vi "Lab Panel V5.10.vi"() -> ()   [LabVIEW 2013] (continued)
                    n2520 = local read "SET LAB01-1"() -> (w4770:T5)
                    n2521 = local read "DISP LAB01-1"() -> (w4771:T4)
                    n2522 = local read "SIG LAB01-1"() -> (w4775:T2)
                    n2523 = Bundle("FAIL LAB01-1"=w4766, "SIG LAB01-1"=w4775, "TEMP START LAB01-1"=w4774, "DISP LAB01-1"=w4771, "SET LAB01-1"=w4770, "TDMS LAB01-1"=w4773) -> (w4760:T32)  [unwired: 1 in]
                    n2524 = call "sub vi - cycle&temp fail v7.vi"("Amps Lo?"=w4772, "Input Cluster"=w4760, "SELECT"=w4769, "Amps Hi?"=w4768, "Result In"=w4763) -> ("(FAIL) out"=w4765:cluster{"FAIL LO":dbl, "FAIL HI":dbl}, "(DISP) out"=w4761:T4, "T-RISE"=w4762:cluster{"T-RISE (L)":dbl, "T-RISE (N)":dbl}, "Result Out"=w4764:bool, "file error"=w4767:errorcluster)  [unwired: 10 in]
                    n2525 = local write "TEMP RISE LAB01-1"(w4762) -> ()
                    n2526 = local write "FAIL LAB01-1"(w4765) -> ()
                    n2527 = local write "DISP LAB01-1"(w4761) -> ()
                    n2528 = local write "RESULT LAB01-1"(w4764) -> ()
                    n2529 = local write "data file error"(w4767) -> ()
                  }
                }
              }
              frame #1 {
                # "LAB01-2"
                n2530 = case shown="True" w4777 {
                  tunnel: w4779 -> [_ w4792]
                  tunnel: w4776 -> [_ w4789]
                  tunnel: w4778 -> [_ w4788]
                  frame False {
                  }
                  frame True {
                    n2531 = local read "TEMP START LAB01-2"() -> (w4794:cluster{"TL":dbl, "TN":dbl})
                    n2532 = local read "FAIL LAB01-2"() -> (w4785:cluster{"LO":dbl, "HI":dbl})
                    n2533 = local read "TDMS LAB01-2"() -> (w4793:refnum<k34>)
                    n2534 = local read "SET LAB01-2"() -> (w4790:T5)
                    n2535 = local read "DISP LAB01-2"() -> (w4791:T4)
                    n2536 = local read "RESULT LAB01-2"() -> (w4782:bool)
                    n2537 = local read "SIG LAB01-2"() -> (w4795:T2)
                    n2538 = Bundle("FAIL LAB01-2"=w4785, "SIG LAB01-2"=w4795, "TEMP START LAB01-2"=w4794, "DISP LAB01-2"=w4791, "SET LAB01-2"=w4790, "TDMS LAB01-2"=w4793) -> (w4780:T33)  [unwired: 1 in]
                    n2539 = call "sub vi - cycle&temp fail v7.vi"("Amps Lo?"=w4792, "Input Cluster"=w4780, "SELECT"=w4789, "Amps Hi?"=w4788, "Result In"=w4782) -> ("(FAIL) out"=w4784:cluster{"FAIL LO":dbl, "FAIL HI":dbl}, "(DISP) out"=w4787:T4, "T-RISE"=w4781:cluster{"T-RISE (L)":dbl, "T-RISE (N)":dbl}, "Result Out"=w4783:bool, "file error"=w4786:errorcluster)  [unwired: 10 in]
                    n2540 = local write "TEMP RISE LAB01-2"(w4781) -> ()
                    n2541 = local write "FAIL LAB01-2"(w4784) -> ()
                    n2542 = local write "DISP LAB01-2"(w4787) -> ()
                    n2543 = local write "RESULT LAB01-2"(w4783) -> ()
                    n2544 = local write "data file error"(w4786) -> ()
                  }
                }
              }
              frame #2 {
                # "LAB02-1"
                n2545 = case shown="True" w4797 {
                  tunnel: w4799 -> [_ w4812]
                  tunnel: w4796 -> [_ w4809]
                  tunnel: w4798 -> [_ w4808]
                  frame False {
                  }
                  frame True {
                    n2546 = local read "TEMP START LAB02-1"() -> (w4814:cluster{"TL":dbl, "TN":dbl})
                    n2547 = local read "FAIL LAB02-1"() -> (w4805:cluster{"LO":dbl, "HI":dbl})
                    n2548 = local read "TDMS LAB02-1"() -> (w4813:refnum<k34>)
                    n2549 = local read "SET LAB02-1"() -> (w4810:T5)
                    n2550 = local read "DISP LAB02-1"() -> (w4811:T4)
                    n2551 = local read "SIG LAB02-1"() -> (w4815:T2)
                    n2552 = local read "RESULT LAB02-1"() -> (w4802:bool)
                    n2553 = Bundle("FAIL LAB02-1"=w4805, "SIG LAB02-1"=w4815, "TEMP START LAB02-1"=w4814, "DISP LAB02-1"=w4811, "SET LAB02-1"=w4810, "TDMS LAB02-1"=w4813) -> (w4800:T34)  [unwired: 1 in]
                    n2554 = call "sub vi - cycle&temp fail v7.vi"("Amps Lo?"=w4812, "Input Cluster"=w4800, "SELECT"=w4809, "Amps Hi?"=w4808, "Result In"=w4802) -> ("(FAIL) out"=w4804:cluster{"FAIL LO":dbl, "FAIL HI":dbl}, "(DISP) out"=w4807:T4, "T-RISE"=w4801:cluster{"T-RISE (L)":dbl, "T-RISE (N)":dbl}, "Result Out"=w4803:bool, "file error"=w4806:errorcluster)  [unwired: 10 in]
                    n2555 = local write "TEMP RISE LAB02-1"(w4801) -> ()
                    n2556 = local write "FAIL LAB02-1"(w4804) -> ()
                    n2557 = local write "DISP LAB02-1"(w4807) -> ()
                    n2558 = local write "RESULT LAB02-1"(w4803) -> ()
                    n2559 = local write "data file error"(w4806) -> ()
                  }
                }
              }
              frame #3 {
                # "LAB02-2"
                n2560 = case shown="True" w4817 {
                  tunnel: w4819 -> [_ w4832]
                  tunnel: w4816 -> [_ w4829]
                  tunnel: w4818 -> [_ w4828]
                  frame False {
                  }
                  frame True {
                    n2561 = local read "TEMP START LAB02-2"() -> (w4834:cluster{"TL":dbl, "TN":dbl})
                    n2562 = local read "FAIL LAB02-2"() -> (w4825:cluster{"LO":dbl, "HI":dbl})
                    n2563 = local read "TDMS LAB02-2"() -> (w4833:refnum<k34>)
                    n2564 = local read "SET LAB02-2"() -> (w4830:T5)
                    n2565 = local read "DISP LAB02-2"() -> (w4831:T4)
                    n2566 = local read "SIG LAB02-2"() -> (w4835:T2)
                    n2567 = local read "RESULT LAB02-2"() -> (w4822:bool)
                    n2568 = Bundle("FAIL LAB02-2"=w4825, "SIG LAB02-2"=w4835, "TEMP START LAB02-2"=w4834, "DISP LAB02-2"=w4831, "SET LAB02-2"=w4830, "TDMS LAB02-2"=w4833) -> (w4820:T35)  [unwired: 1 in]
                    n2569 = call "sub vi - cycle&temp fail v7.vi"("Amps Lo?"=w4832, "Input Cluster"=w4820, "SELECT"=w4829, "Amps Hi?"=w4828, "Result In"=w4822) -> ("(FAIL) out"=w4824:cluster{"FAIL LO":dbl, "FAIL HI":dbl}, "(DISP) out"=w4827:T4, "T-RISE"=w4821:cluster{"T-RISE (L)":dbl, "T-RISE (N)":dbl}, "Result Out"=w4823:bool, "file error"=w4826:errorcluster)  [unwired: 10 in]
                    n2570 = local write "TEMP RISE LAB02-2"(w4821) -> ()
                    n2571 = local write "FAIL LAB02-2"(w4824) -> ()
                    n2572 = local write "DISP LAB02-2"(w4827) -> ()
                    n2573 = local write "RESULT LAB02-2"(w4823) -> ()
                    n2574 = local write "data file error"(w4826) -> ()
                  }
                }
              }
              frame #4 {
                # "LAB03-1"
                n2575 = case shown="True" w4837 {
                  tunnel: w4839 -> [_ w4852]
                  tunnel: w4836 -> [_ w4849]
                  tunnel: w4838 -> [_ w4848]
                  frame False {
                  }
                  frame True {
                    n2576 = local read "TEMP START LAB03-1"() -> (w4854:cluster{"TL":dbl, "TN":dbl})
                    n2577 = local read "FAIL LAB03-1"() -> (w4845:cluster{"LO":dbl, "HI":dbl})
                    n2578 = local read "TDMS LAB03-1"() -> (w4853:refnum<k34>)
                    n2579 = local read "SET LAB03-1"() -> (w4850:T5)
                    n2580 = local read "DISP LAB03-1"() -> (w4851:T4)
                    n2581 = local read "SIG LAB03-1"() -> (w4855:T2)
                    n2582 = local read "RESULT LAB03-1"() -> (w4842:bool)
                    n2583 = Bundle("FAIL LAB03-1"=w4845, "SIG LAB03-1"=w4855, "TEMP START LAB03-1"=w4854, "DISP LAB03-1"=w4851, "SET LAB03-1"=w4850, "TDMS LAB03-1"=w4853) -> (w4840:T36)  [unwired: 1 in]
                    n2584 = call "sub vi - cycle&temp fail v7.vi"("Amps Lo?"=w4852, "Input Cluster"=w4840, "SELECT"=w4849, "Amps Hi?"=w4848, "Result In"=w4842) -> ("(FAIL) out"=w4844:cluster{"FAIL LO":dbl, "FAIL HI":dbl}, "(DISP) out"=w4847:T4, "T-RISE"=w4841:cluster{"T-RISE (L)":dbl, "T-RISE (N)":dbl}, "Result Out"=w4843:bool, "file error"=w4846:errorcluster)  [unwired: 10 in]
                    n2585 = local write "TEMP RISE LAB03-1"(w4841) -> ()
                    n2586 = local write "FAIL LAB03-1"(w4844) -> ()
                    n2587 = local write "DISP LAB03-1"(w4847) -> ()
                    n2588 = local write "RESULT LAB03-1"(w4843) -> ()
                    n2589 = local write "data file error"(w4846) -> ()
                  }
                }
              }
              frame #5 {
                # "LAB03-2"
                n2590 = case shown="True" w4857 {
                  tunnel: w4859 -> [_ w4872]
                  tunnel: w4856 -> [_ w4869]
                  tunnel: w4858 -> [_ w4868]
                  frame False {
                  }
                  frame True {
                    n2591 = local read "TEMP START LAB03-2"() -> (w4874:cluster{"TL":dbl, "TN":dbl})
                    n2592 = local read "FAIL LAB03-2"() -> (w4865:cluster{"LO":dbl, "HI":dbl})
                    n2593 = local read "TDMS LAB03-2"() -> (w4873:refnum<k34>)
                    n2594 = local read "SET LAB03-2"() -> (w4870:T5)
                    n2595 = local read "DISP LAB03-2"() -> (w4871:T4)
                    n2596 = local read "RESULT LAB03-2"() -> (w4862:bool)
                    n2597 = local read "SIG LAB03-2"() -> (w4875:T2)
                    n2598 = Bundle("FAIL LAB03-2"=w4865, "SIG LAB03-2"=w4875, "TEMP START LAB03-2"=w4874, "DISP LAB03-2"=w4871, "SET LAB03-2"=w4870, "TDMS LAB03-2"=w4873) -> (w4860:T37)  [unwired: 1 in]
                    n2599 = call "sub vi - cycle&temp fail v7.vi"("Amps Lo?"=w4872, "Input Cluster"=w4860, "SELECT"=w4869, "Amps Hi?"=w4868, "Result In"=w4862) -> ("(FAIL) out"=w4864:cluster{"FAIL LO":dbl, "FAIL HI":dbl}, "(DISP) out"=w4867:T4, "T-RISE"=w4861:cluster{"T-RISE (L)":dbl, "T-RISE (N)":dbl}, "Result Out"=w4863:bool, "file error"=w4866:errorcluster)  [unwired: 10 in]
                    n2600 = local write "FAIL LAB03-2"(w4864) -> ()
                    n2601 = local write "TEMP RISE LAB03-2"(w4861) -> ()
                    n2602 = local write "DISP LAB03-2"(w4867) -> ()
                    n2603 = local write "RESULT LAB03-2"(w4863) -> ()
                    n2604 = local write "data file error"(w4866) -> ()
                  }
                }
              }
              frame #6 {
                # "LAB04-1"
                n2605 = case shown="True" w4877 {
                  tunnel: w4879 -> [_ w4892]
                  tunnel: w4876 -> [_ w4889]
                  tunnel: w4878 -> [_ w4888]
                  frame False {
                  }
                  frame True {
                    n2606 = local read "TEMP START LAB04-1"() -> (w4894:cluster{"TL":dbl, "TN":dbl})
                    n2607 = local read "FAIL LAB04-1"() -> (w4885:cluster{"LO":dbl, "HI":dbl})
                    n2608 = local read "TDMS LAB04-1"() -> (w4893:refnum<k34>)
                    n2609 = local read "SET LAB04-1"() -> (w4890:T5)
                    n2610 = local read "DISP LAB04-1"() -> (w4891:T4)
                    n2611 = local read "SIG LAB04-1"() -> (w4895:T2)
                    n2612 = local read "RESULT LAB04-1"() -> (w4882:bool)
                    n2613 = Bundle("FAIL LAB04-1"=w4885, "SIG LAB04-1"=w4895, "TEMP START LAB04-1"=w4894, "DISP LAB04-1"=w4891, "SET LAB04-1"=w4890, "TDMS LAB04-1"=w4893) -> (w4880:T38)  [unwired: 1 in]
                    n2614 = call "sub vi - cycle&temp fail v7.vi"("Amps Lo?"=w4892, "Input Cluster"=w4880, "SELECT"=w4889, "Amps Hi?"=w4888, "Result In"=w4882) -> ("(FAIL) out"=w4884:cluster{"FAIL LO":dbl, "FAIL HI":dbl}, "(DISP) out"=w4887:T4, "T-RISE"=w4881:cluster{"T-RISE (L)":dbl, "T-RISE (N)":dbl}, "Result Out"=w4883:bool, "file error"=w4886:errorcluster)  [unwired: 10 in]
                    n2615 = local write "TEMP RISE LAB04-1"(w4881) -> ()
                    n2616 = local write "FAIL LAB04-1"(w4884) -> ()
                    n2617 = local write "DISP LAB04-1"(w4887) -> ()
                    n2618 = local write "RESULT LAB04-1"(w4883) -> ()
                    n2619 = local write "data file error"(w4886) -> ()
                  }
                }
              }
              frame #7 {
                # "LAB04-2"
                n2620 = case shown="True" w4897 {
                  tunnel: w4899 -> [_ w4912]
                  tunnel: w4896 -> [_ w4909]
                  tunnel: w4898 -> [_ w4908]
                  frame False {
                  }
                  frame True {
                    n2621 = local read "TEMP START LAB04-2"() -> (w4914:cluster{"TL":dbl, "TN":dbl})
                    n2622 = local read "FAIL LAB04-2"() -> (w4905:cluster{"LO":dbl, "HI":dbl})
                    n2623 = local read "TDMS LAB04-2"() -> (w4913:refnum<k34>)
                    n2624 = local read "SET LAB04-2"() -> (w4910:T5)
                    n2625 = local read "DISP LAB04-2"() -> (w4911:T4)
                    n2626 = local read "SIG LAB04-2"() -> (w4915:T2)
                    n2627 = local read "RESULT LAB04-2"() -> (w4902:bool)
                    n2628 = Bundle("FAIL LAB04-2"=w4905, "SIG LAB04-2"=w4915, "TEMP START LAB04-2"=w4914, "DISP LAB04-2"=w4911, "SET LAB04-2"=w4910, "TDMS LAB04-2"=w4913) -> (w4900:T39)  [unwired: 1 in]
                    n2629 = call "sub vi - cycle&temp fail v7.vi"("Amps Lo?"=w4912, "Input Cluster"=w4900, "SELECT"=w4909, "Amps Hi?"=w4908, "Result In"=w4902) -> ("(FAIL) out"=w4904:cluster{"FAIL LO":dbl, "FAIL HI":dbl}, "(DISP) out"=w4907:T4, "T-RISE"=w4901:cluster{"T-RISE (L)":dbl, "T-RISE (N)":dbl}, "Result Out"=w4903:bool, "file error"=w4906:errorcluster)  [unwired: 10 in]
                    n2630 = local write "TEMP RISE LAB04-2"(w4901) -> ()
                    n2631 = local write "FAIL LAB04-2"(w4904) -> ()
                    n2632 = local write "DISP LAB04-2"(w4907) -> ()
                    n2633 = local write "RESULT LAB04-2"(w4903) -> ()
                    n2634 = local write "data file error"(w4906) -> ()
                  }
                }
              }
              frame #8 {
                # "LAB05-1"
                n2635 = case shown="True" w4917 {
                  tunnel: w4919 -> [_ w4932]
                  tunnel: w4916 -> [_ w4929]
                  tunnel: w4918 -> [_ w4928]
                  frame False {
                  }
                  frame True {
                    n2636 = local read "TEMP START LAB05-1"() -> (w4934:cluster{"TL":dbl, "TN":dbl})
                    n2637 = local read "FAIL LAB05-1"() -> (w4925:cluster{"LO":dbl, "HI":dbl})
                    n2638 = local read "TDMS LAB05-1"() -> (w4933:refnum<k34>)
                    n2639 = local read "SET LAB05-1"() -> (w4930:T5)
                    n2640 = local read "DISP LAB05-1"() -> (w4931:T4)
                    n2641 = local read "SIG LAB05-1"() -> (w4935:T2)
                    n2642 = local read "RESULT LAB05-1"() -> (w4922:bool)
                    n2643 = Bundle("FAIL LAB05-1"=w4925, "SIG LAB05-1"=w4935, "TEMP START LAB05-1"=w4934, "DISP LAB05-1"=w4931, "SET LAB05-1"=w4930, "TDMS LAB05-1"=w4933) -> (w4920:T40)  [unwired: 1 in]
                    n2644 = call "sub vi - cycle&temp fail v7.vi"("Amps Lo?"=w4932, "Input Cluster"=w4920, "SELECT"=w4929, "Amps Hi?"=w4928, "Result In"=w4922) -> ("(FAIL) out"=w4924:cluster{"FAIL LO":dbl, "FAIL HI":dbl}, "(DISP) out"=w4927:T4, "T-RISE"=w4921:cluster{"T-RISE (L)":dbl, "T-RISE (N)":dbl}, "Result Out"=w4923:bool, "file error"=w4926:errorcluster)  [unwired: 10 in]
                    n2645 = local write "TEMP RISE LAB05-1"(w4921) -> ()
                    n2646 = local write "FAIL LAB05-1"(w4924) -> ()
                    n2647 = local write "DISP LAB05-1"(w4927) -> ()
                    n2648 = local write "RESULT LAB05-1"(w4923) -> ()
                    n2649 = local write "data file error"(w4926) -> ()
                  }
                }
              }
              frame #9 {
                # "LAB05-2"
                n2650 = case shown="True" w4937 {
                  tunnel: w4939 -> [_ w4952]
                  tunnel: w4936 -> [_ w4949]
                  tunnel: w4938 -> [_ w4948]
                  frame False {
                  }
                  frame True {
                    n2651 = local read "TEMP START LAB05-2"() -> (w4954:cluster{"TL":dbl, "TN":dbl})
                    n2652 = local read "FAIL LAB05-2"() -> (w4945:cluster{"LO":dbl, "HI":dbl})
                    n2653 = local read "TDMS LAB05-2"() -> (w4953:refnum<k34>)
                    n2654 = local read "SET LAB05-2"() -> (w4950:T5)
                    n2655 = local read "DISP LAB05-2"() -> (w4951:T4)
                    n2656 = local read "SIG LAB05-2"() -> (w4955:T2)
                    n2657 = local read "RESULT LAB05-2"() -> (w4942:bool)
                    n2658 = Bundle("FAIL LAB05-2"=w4945, "SIG LAB05-2"=w4955, "TEMP START LAB05-2"=w4954, "DISP LAB05-2"=w4951, "SET LAB05-2"=w4950, "TDMS LAB05-2"=w4953) -> (w4940:T41)  [unwired: 1 in]
                    n2659 = call "sub vi - cycle&temp fail v7.vi"("Amps Lo?"=w4952, "Input Cluster"=w4940, "SELECT"=w4949, "Amps Hi?"=w4948, "Result In"=w4942) -> ("(FAIL) out"=w4944:cluster{"FAIL LO":dbl, "FAIL HI":dbl}, "(DISP) out"=w4947:T4, "T-RISE"=w4941:cluster{"T-RISE (L)":dbl, "T-RISE (N)":dbl}, "Result Out"=w4943:bool, "file error"=w4946:errorcluster)  [unwired: 10 in]
                    n2660 = local write "TEMP RISE LAB05-2"(w4941) -> ()
                    n2661 = local write "FAIL LAB05-2"(w4944) -> ()
                    n2662 = local write "DISP LAB05-2"(w4947) -> ()
                    n2663 = local write "RESULT LAB05-2"(w4943) -> ()
                    n2664 = local write "data file error"(w4946) -> ()
                  }
                }
              }
            }
          }
          frame #15 {
            # "run calibration routine"
            n2665 = local read "SET (cal)"() -> (w4956:bool)
            n2666 = case shown="True" w4956 {
              frame False {
              }
              frame True {
                n2667 = stacked-sequence {
                  seq-local: [w4957 _ _] -> [_ w4959 _]
                  frame #0 {
                    n2668 = call "CALIBRATION PASSWORD"() -> ("PASSWORD"=w4957:string)  [unwired: 17 in, 2 out]
                  }
                  frame #1 {
                    n2669 = Equal?(x=w4959, y="7777") -> (x = y?=w4958:bool)
                    n2670 = case shown="True" w4958 {
                      frame False {
                      }
                      frame True {
                        n2671 = stacked-sequence {
                          frame #0 {
                            n2672 = local read "Temp Test Cal"() -> (w4961:dbl)
                            n2673 = call "sub vi - calibration v1.vi"("Temp Test Cal"=w4961) -> ()  [unwired: 11 in]
                          }
                          frame #1 {
                            n2674 = call "sub vi - get calibration values v1.vi"() -> ("TEMP REF CAL"=w4962:dbl, "LAB01 (CAL)"=w4967:T14, "LAB02 (CAL)"=w4966:T15, "LAB03 (CAL)"=w4965:T14, "LAB04 (CAL)"=w4964:T14, "calibration file error out"=w4968:errorcluster, "LAB05 (CAL)"=w4963:T14)  [unwired: 9 in]
                            n2675 = local write "TEMP REF cal"(w4962) -> ()
                            n2676 = local write "cal file error out"(w4968) -> ()
                            n2677 = local write "CAL LAB04"(w4964) -> ()
                            n2678 = local write "CAL LAB05"(w4963) -> ()
                            n2679 = local write "CAL LAB01"(w4967) -> ()
                            n2680 = local write "CAL LAB02"(w4966) -> ()
                            n2681 = local write "CAL LAB03"(w4965) -> ()
                          }
                        }
                      }
                    }
                  }
                  frame #2 {
                    n2682 = local write "SET (cal)"(FALSE) -> ()
                  }
                }
              }
            }
          }
          frame #16 {
            # "save certain settings to file"
            n2683 = String To Path(string="c:\\crabtree\\Set Up\\") -> (path=w4971:path)
            n2684 = Build Path(base path=w4971, name or relative path="settings.bin") -> (appended path=w4973:path)
            n2685 = Build Path(base path=w4971, name or relative path="mail.bin") -> (appended path=w4970:path)
            n2686 = Create Folder(path (use dialog)=w4971) -> (error out=w4976:errorcluster)  [unwired: 2 in, 2 out]
            n2687 = call <vilib>:"Clear Errors.vi"("error in (no error)"=w4976) -> ()  [unwired: 6 in, 1 out]
            n2688 = stacked-sequence {
              seq-local: [w4988 _] -> [_ w5001]
              tunnel: w4973 -> [_ w5002]
              tunnel: w4970 -> [_ w5000]
              frame #0 {
                n2689 = local read "C drive data root dir"() -> (w4987:path)
                n2690 = local read "Select COM port"() -> (w4984:refnum<visa-resource-name>)
                n2691 = local read "Network Directory"() -> (w4993:path)
                n2692 = local read "SET LAB05-2"() -> (w4992:T5)
                n2693 = local read "SET LAB05-1"() -> (w4991:T5)
                n2694 = local read "SET LAB04-2"() -> (w4990:T5)
                n2695 = local read "SET LAB03-2"() -> (w4994:T5)
                n2696 = local read "SET LAB04-1"() -> (w4989:T5)
                n2697 = local read "SET LAB03-1"() -> (w4995:T5)
                n2698 = local read "SET LAB02-2"() -> (w4996:T5)
                n2699 = local read "SET LAB02-1"() -> (w4997:T5)
                n2700 = local read "Temp Delay Lps"() -> (w4983:dbl)
                n2701 = local read "Amps Fail level"() -> (w4979:dbl)
                n2702 = local read "SET LAB01-2"() -> (w4998:T5)
                n2703 = local read "Temp Test Cal"() -> (w4980:dbl)
                n2704 = local read "SET LAB01-1"() -> (w4999:T5)
                n2705 = local read "Mail Test File To:"() -> (w4978:string)
                n2706 = local read "Temp Value"() -> (w4982:dbl)
                n2707 = local read "Fail Loops"() -> (w4981:dbl)
                n2708 = local read "Mail Test Fail"() -> (w4977:bool)
                n2709 = local read "RATE (Hz)"() -> (w4986:dbl)
                n2710 = local read "SAMPLES"() -> (w4985:dbl)
                n2711 = Bundle("SET LAB01-1"=w4999, "SET LAB01-2"=w4998, "SET LAB02-1"=w4997, "SET LAB02-2"=w4996, "SET LAB03-1"=w4995, "SET LAB03-2"=w4994, "SET LAB04-1"=w4989, "SET LAB04-2"=w4990, "SET LAB05-1"=w4991, "SET LAB05-2"=w4992, "Network Directory"=w4993, "C drive data root dir"=w4987, "RATE (Hz)"=w4986, "SAMPLES"=w4985, "Select COM port"=w4984, "Temp Delay Lps"=w4983, "Temp Value"=w4982, "Fail Loops"=w4981, "Temp Test Cal"=w4980, "Amps Fail level"=w4979, "Mail Test File To:"=w4978, "Mail Test Fail"=w4977) -> (w4988:T22)  [unwired: 1 in]
              }
              frame #1 {
                n2712 = event shown="[1] \"SET LAB01-1\", \"SET LAB01-2\", \"SET LAB02-1\", \"SET LAB02-2\", \"SET LAB03-1\", \"SET LAB03-2\", \"SET LAB04-1\", \"SET LAB04-2\", \"SET LAB05-1\", \"SET LAB05-2\", \"Network Directory\", \"C drive data root dir\", \"RATE (Hz)\", \"SAMPLES\", \"Select COM port\", \"Temp Delay Lps\", \"Temp Value\", \"Fail Loops\", \"Temp Test Cal\", \"Amps Fail level\", \"Mail Test File To:\", \"Mail Test Fail\": Value Change" {
                  selector: _ -> [_ _ _]
                  dyn-events: _ -> [_ _ _]
                  timeout: 10.0 -> [_ _ _]
                  tunnel: w5002 -> [_ w5004 _]
                  tunnel: w5001 -> [_ w5005 _]
                  tunnel: w5000 -> [_ _ w5016]
                  event Timeout {
                    n2713 = event-data() -> ()  [unwired: 1 in, 3 out]
                  }
                  event "SET LAB01-1", "SET LAB01-2", "SET LAB02-1", "SET LAB02-2", "SET LAB03-1", "SET LAB03-2", "SET LAB04-1", "SET LAB04-2", "SET LAB05-1", "SET LAB05-2", "Network Directory", "C drive data root dir", "RATE (Hz)", "SAMPLES", "Select COM port", "Temp Delay Lps", "Temp Value", "Fail Loops", "Temp Test Cal", "Amps Fail level", "Mail Test File To:", "Mail Test Fail": Value Change {
                    n2714 = event-data() -> ()  [unwired: 1 in, 6 out]
                    n2715 = Open/Create/Replace File(file path (use dialog)=w5004, operation (0:open)=T21."replace or create") -> (refnum out=w5010:refnum<file>, error out=w5009:errorcluster)  [unwired: 4 in, 1 out]
                    n2716 = Write to Binary File(file (use dialog)=w5010, data=w5005, error in=w5009) -> (refnum out=w5008:refnum<file>, error out=w5007:errorcluster)  [unwired: 3 in, 1 out]
                    n2717 = Close File(refnum=w5008, error in=w5007) -> (error out=w5006:errorcluster)  [unwired: 1 out]
                    n2718 = local write "data file error"(w5006) -> ()
                  }
                  event "MAIL SETTINGS.OUT SERVER ADDRESS", "MAIL SETTINGS.FROM ACCOUNT", "MAIL SETTINGS.USER NAME", "MAIL SETTINGS.PASSWORD", "Auto Mail Send", "TO (string):": Value Change {
                    n2719 = event-data() -> ()  [unwired: 1 in, 6 out]
                    n2720 = local read "MAIL SETTINGS"() -> (w5015:T7)
                    n2721 = local read "Auto Mail Send"() -> (w5013:bool)
                    n2722 = local read "TO (string):"() -> (w5012:string)
                    n2723 = Open/Create/Replace File(file path (use dialog)=w5016, operation (0:open)=T21."replace or create") -> (refnum out=w5021:refnum<file>, error out=w5020:errorcluster)  [unwired: 4 in, 1 out]
                    n2724 = Bundle("MAIL SETTINGS"=w5015, "Auto Mail Send"=w5013, "TO (string):"=w5012) -> (w5014:T42)  [unwired: 1 in]
                    n2725 = Write to Binary File(file (use dialog)=w5021, data=w5014, error in=w5020) -> (refnum out=w5019:refnum<file>, error out=w5018:errorcluster)  [unwired: 3 in, 1 out]
                    n2726 = Close File(refnum=w5019, error in=w5018) -> (error out=w5017:errorcluster)  [unwired: 1 out]
                    n2727 = local write "data file error"(w5017) -> ()
                  }
                }
              }
            }
          }
          frame #17 {
            # "mail control"
            n2728 = local read "MAIL SETTINGS"() -> (w5038:T7)
            n2729 = local read "Auto Mail Send"() -> (w5024:bool)
            n2730 = Unbundle(w5038) -> ("OUT SERVER ADDRESS"=w5037:string, "FROM ACCOUNT"=w5036:string, "TEST MAIL"=w5035:bool)  [unwired: 4 out]
            n2731 = stacked-sequence {
              tunnel: "TO (string):" -> [_ w5077]
              tunnel: w5038 -> [w5043 w5076]
              tunnel: w5037 -> [w5042 w5075]
              tunnel: w5036 -> [w5041 w5074]
              tunnel: w5035 -> [w5040 _]
              tunnel: w5024 -> [_ w5073]
              tunnel: w5034 -> [_ w5072]
              tunnel: w5033 -> [_ w5071]
              tunnel: w5032 -> [_ w5070]
              tunnel: w5031 -> [_ w5069]
              tunnel: w5030 -> [_ w5068]
              tunnel: w5029 -> [_ w5067]
              tunnel: w5028 -> [_ w5066]
              tunnel: w5027 -> [_ w5065]
              tunnel: w5026 -> [_ w5064]
              tunnel: w5025 -> [_ w5063]
              tunnel: "TO (string):" -> [w5039 _]
              frame #0 {
                # "mail test"
                n2732 = case shown="True" w5040 {
                  tunnel: w5043 -> [_ w5047]
                  tunnel: w5039 -> [_ w5046]
                  tunnel: w5042 -> [_ w5045]
                  tunnel: w5041 -> [_ w5044]
                  frame False {
                  }
                  frame True {
                    n2733 = stacked-sequence {
                      seq-local: [_ _ w5057 _] -> [_ _ _ w5058]
                      tunnel: w5047 -> [w5050 _ _ w5062]
                      tunnel: w5046 -> [_ _ w5055 _]
                      tunnel: w5045 -> [_ _ w5053 _]
                      tunnel: w5044 -> [_ _ w5054 _]
                      frame #0 {
                        n2734 = Bundle(cluster=w5050, "TEST MAIL STATUS"="TEST START") -> (w5048:T7)  [unwired: 6 in]
                        n2735 = local write "MAIL SETTINGS"(w5048) -> ()
                      }
                      frame #1 {
                        n2736 = Wait (ms)(milliseconds to wait=500) -> ()  [unwired: 1 out]
                      }
                      frame #2 {
                        n2737 = call "sub vi - send mail v5.vi"("TO:"=w5055, "subject"="MAIL TEST FROM LAB PANEL", "from"=w5054, "out going server"=w5053, "message"="TEST MESSAGE") -> ("error out"=w5057:errorcluster)  [unwired: 10 in]
                      }
                      frame #3 {
                        n2738 = Bundle(cluster=w5062, "TEST MAIL"=FALSE, "TEST MAIL STATUS"="TEST END", "mail error"=w5058) -> (w5060:T7)  [unwired: 4 in]
                        n2739 = local write "MAIL SETTINGS"(w5060) -> ()
                      }
                    }
                  }
                }
              }
              frame #1 {
                # "mail report"
                n2740 = stacked-sequence {
                  seq-local: [_ w5120 _ _] -> [_ _ _ w5310]
                  seq-local: [_ _ w5223 _] -> [_ _ _ w5300]
                  seq-local: [w5087 _ _ _] -> [_ w5137 _ _]
                  seq-local: [w5086 _ _ _] -> [_ w5136 _ _]
                  seq-local: [w5084 _ _ _] -> [_ w5134 _ _]
                  seq-local: [w5085 _ _ _] -> [_ w5135 _ _]
                  seq-local: [w5083 _ _ _] -> [_ w5133 _ _]
                  seq-local: [w5082 _ _ _] -> [_ w5128 _ _]
                  seq-local: [w5081 _ _ _] -> [_ w5129 _ _]
                  seq-local: [w5080 _ _ _] -> [_ w5130 _ _]
                  seq-local: [w5079 _ _ _] -> [_ w5131 _ _]
                  seq-local: [w5078 _ _ _] -> [_ w5132 _ _]
                  tunnel: w5077 -> [_ _ _ w5311]
                  tunnel: w5076 -> [_ _ _ w5294]
                  tunnel: w5075 -> [_ _ _ w5308]
                  tunnel: w5074 -> [_ _ _ w5307]
                  tunnel: w5073 -> [w5118 _ _ w5302]
                  tunnel: w5072 -> [_ _ w5253 _]
                  tunnel: w5071 -> [_ _ w5250 _]
                  tunnel: w5070 -> [_ _ w5249 _]
                  tunnel: w5069 -> [_ _ w5248 _]
                  tunnel: w5068 -> [_ _ w5247 _]
                  tunnel: w5067 -> [_ _ w5246 _]
                  tunnel: w5066 -> [_ _ w5245 _]
                  tunnel: w5065 -> [_ _ w5244 _]
                  tunnel: w5064 -> [_ _ w5243 _]
                  tunnel: w5063 -> [_ _ w5242 _]
                  frame #0 {
                    n2741 = case shown="False" w5118 {
                      frame False {
                        n2742 = local write "mail control"("") -> ()
                      }
                      frame True {
                      }
                    }
                    n2743 = local read "SET LAB01-1"() -> (w5117:T5)
                    n2744 = local read "SET LAB01-2"() -> (w5116:T5)
                    n2745 = local read "SET LAB02-1"() -> (w5115:T5)
                    n2746 = local read "SET LAB02-2"() -> (w5114:T5)
                    n2747 = local read "SET LAB03-1"() -> (w5113:T5)
                    n2748 = local read "SET LAB04-1"() -> (w5111:T5)
                    n2749 = local read "SET LAB05-1"() -> (w5109:T5)
                    n2750 = local read "SET LAB03-2"() -> (w5112:T5)
                    n2751 = local read "SET LAB04-2"() -> (w5110:T5)
                    n2752 = local read "SET LAB05-2"() -> (w5108:T5)
                    n2753 = Unbundle(w5113) -> ("DESCRIPTION"=w5093:string)  [unwired: 4 out]
                    n2754 = Unbundle(w5112) -> ("DESCRIPTION"=w5092:string)  [unwired: 4 out]
                    n2755 = Unbundle(w5111) -> ("DESCRIPTION"=w5091:string)  [unwired: 4 out]
                    n2756 = Unbundle(w5108) -> ("DESCRIPTION"=w5088:string)  [unwired: 4 out]
                    n2757 = Unbundle(w5114) -> ("DESCRIPTION"=w5094:string)  [unwired: 4 out]
                    n2758 = Unbundle(w5110) -> ("DESCRIPTION"=w5090:string)  [unwired: 4 out]
                    n2759 = Unbundle(w5117) -> ("DESCRIPTION"=w5106:string)  [unwired: 4 out]
                    n2760 = Unbundle(w5115) -> ("DESCRIPTION"=w5095:string)  [unwired: 4 out]
                    n2761 = Unbundle(w5109) -> ("DESCRIPTION"=w5089:string)  [unwired: 4 out]
                    n2762 = Unbundle(w5116) -> ("DESCRIPTION"=w5096:string)  [unwired: 4 out]
                    n2763 = Concatenate Strings("[LAB05-2/", w5088) -> (w5078:string)
                    n2764 = Concatenate Strings("[LAB05-1/", w5089) -> (w5079:string)
                    n2765 = Concatenate Strings("[LAB04-2/", w5090) -> (w5080:string)
                    n2766 = Concatenate Strings("[LAB03-2/", w5092) -> (w5082:string)
                    n2767 = Concatenate Strings("[LAB04-1/", w5091) -> (w5081:string)
                    n2768 = Concatenate Strings("[LAB03-1/", w5093) -> (w5083:string)
                    n2769 = Concatenate Strings("[LAB01-2/", w5096) -> (w5086:string)
                    n2770 = Concatenate Strings("[LAB02-2/", w5094) -> (w5084:string)
                    n2771 = Concatenate Strings("[LAB01-1/", w5106) -> (w5087:string)
                    n2772 = Concatenate Strings("[LAB02-1/", w5095) -> (w5085:string)
                  }
                  frame #1 {
                    w5141 = "/"
                    w5142 = 2.0
                    n2773 = local read "DISP LAB01-2"() -> (w5221:T4)
                    n2774 = local read "DISP LAB01-1"() -> (w5222:T4)
                    n2775 = local read "DISP LAB02-1"() -> (w5220:T4)
                    n2776 = local read "DISP LAB03-2"() -> (w5217:T4)
                    n2777 = local read "DISP LAB02-2"() -> (w5219:T4)
                    n2778 = local read "DISP LAB03-1"() -> (w5218:T4)
                    n2779 = local read "DISP LAB04-2"() -> (w5215:T4)
                    n2780 = local read "DISP LAB04-1"() -> (w5216:T4)
                    n2781 = local read "DISP LAB05-1"() -> (w5214:T4)
                    n2782 = local read "DISP LAB05-2"() -> (w5213:T4)
                    n2783 = Unbundle(w5221) -> ("CYCLE"=w5205:dbl, "MINS"=w5204:dbl, "STATUS"=w5201:string)
                    n2784 = Unbundle(w5222) -> ("CYCLE"=w5210:dbl, "MINS"=w5209:dbl, "STATUS"=w5206:string)
                    n2785 = Unbundle(w5220) -> ("CYCLE"=w5198:dbl, "MINS"=w5197:dbl, "STATUS"=w5196:string)
                    n2786 = Unbundle(w5217) -> ("CYCLE"=w5185:dbl, "MINS"=w5184:dbl, "STATUS"=w5181:string)
                    n2787 = Unbundle(w5218) -> ("CYCLE"=w5190:dbl, "MINS"=w5189:dbl, "STATUS"=w5186:string)
                    n2788 = Unbundle(w5219) -> ("CYCLE"=w5195:dbl, "MINS"=w5194:dbl, "STATUS"=w5191:string)
                    n2789 = Unbundle(w5216) -> ("CYCLE"=w5180:dbl, "MINS"=w5179:dbl, "STATUS"=w5176:string)
                    n2790 = Unbundle(w5215) -> ("CYCLE"=w5175:dbl, "MINS"=w5174:dbl, "STATUS"=w5171:string)
                    n2791 = Unbundle(w5214) -> ("CYCLE"=w5170:dbl, "MINS"=w5169:dbl, "STATUS"=w5166:string)
                    n2792 = Unbundle(w5213) -> ("CYCLE"=w5212:dbl, "MINS"=w5211:dbl, "STATUS"=w5163:string)
                    n2793 = Number To Decimal String(number=w5198) -> (decimal integer string=w5200:string)  [unwired: 1 in]
                    n2794 = Number To Decimal String(number=w5195) -> (decimal integer string=w5193:string)  [unwired: 1 in]
                    n2795 = Number To Decimal String(number=w5190) -> (decimal integer string=w5188:string)  [unwired: 1 in]
                    n2796 = Number To Decimal String(number=w5205) -> (decimal integer string=w5203:string)  [unwired: 1 in]
                    n2797 = Number To Decimal String(number=w5185) -> (decimal integer string=w5183:string)  [unwired: 1 in]
                    n2798 = Number To Decimal String(number=w5210) -> (decimal integer string=w5208:string)  [unwired: 1 in]
                    n2799 = Number To Decimal String(number=w5212) -> (decimal integer string=w5165:string)  [unwired: 1 in]
                    n2800 = Number To Decimal String(number=w5180) -> (decimal integer string=w5178:string)  [unwired: 1 in]
                    n2801 = Number To Decimal String(number=w5175) -> (decimal integer string=w5173:string)  [unwired: 1 in]
                    n2802 = Number To Decimal String(number=w5170) -> (decimal integer string=w5168:string)  [unwired: 1 in]
                    n2803 = Number To Fractional String(number=w5197, precision (6)=w5142) -> (F-format string=w5199:string)  [unwired: 2 in]
                    n2804 = Number To Fractional String(number=w5184, precision (6)=w5142) -> (F-format string=w5182:string)  [unwired: 2 in]
                    n2805 = Number To Fractional String(number=w5194, precision (6)=w5142) -> (F-format string=w5192:string)  [unwired: 2 in]
                    n2806 = Number To Fractional String(number=w5189, precision (6)=w5142) -> (F-format string=w5187:string)  [unwired: 2 in]
                    n2807 = Number To Fractional String(number=w5174, precision (6)=w5142) -> (F-format string=w5172:string)  [unwired: 2 in]
                    n2808 = Number To Fractional String(number=w5179, precision (6)=w5142) -> (F-format string=w5177:string)  [unwired: 2 in]
                    n2809 = Number To Fractional String(number=w5204, precision (6)=w5142) -> (F-format string=w5202:string)  [unwired: 2 in]
                    n2810 = Number To Fractional String(number=w5169, precision (6)=w5142) -> (F-format string=w5167:string)  [unwired: 2 in]
                    n2811 = Number To Fractional String(number=w5209, precision (6)=w5142) -> (F-format string=w5207:string)  [unwired: 2 in]
                    n2812 = Number To Fractional String(number=w5211, precision (6)=w5142) -> (F-format string=w5164:string)  [unwired: 2 in]
                    n2813 = Concatenate Strings(w5141, w5183, w5141, w5182, w5141, w5181) -> (w5157:string)
                    n2814 = Concatenate Strings(w5141, w5178, w5141, w5177, w5141, w5176) -> (w5156:string)
                    n2815 = Concatenate Strings(w5141, w5173, w5141, w5172, w5141, w5171) -> (w5155:string)
                    n2816 = Concatenate Strings(w5141, w5168, w5141, w5167, w5141, w5166) -> (w5154:string)
                    n2817 = Concatenate Strings(w5141, w5165, w5141, w5164, w5141, w5163) -> (w5153:string)
                    n2818 = Concatenate Strings(w5141, w5208, w5141, w5207, w5141, w5206) -> (w5162:string)
                    n2819 = Concatenate Strings(w5141, w5188, w5141, w5187, w5141, w5186) -> (w5158:string)
                    n2820 = Concatenate Strings(w5141, w5203, w5141, w5202, w5141, w5201) -> (w5161:string)
                    n2821 = Concatenate Strings(w5141, w5200, w5141, w5199, w5141, w5196) -> (w5160:string)
                    n2822 = Concatenate Strings(w5141, w5193, w5141, w5192, w5141, w5191) -> (w5159:string)
                    n2823 = Concatenate Strings("]", "\r") -> (w5138:string)
                    n2824 = Concatenate Strings(w5133, w5158, w5138) -> (w5148:string)
                    n2825 = Concatenate Strings(w5135, w5160, w5138) -> (w5150:string)
                    n2826 = Concatenate Strings(w5134, w5159, w5138) -> (w5149:string)
                    n2827 = Concatenate Strings(w5130, w5155, w5138) -> (w5145:string)
                    n2828 = Concatenate Strings(w5131, w5154, w5138) -> (w5146:string)
                    n2829 = Concatenate Strings(w5129, w5156, w5138) -> (w5144:string)
                    n2830 = Concatenate Strings(w5128, w5157, w5138) -> (w5143:string)
                    n2831 = Concatenate Strings(w5132, w5153, w5138) -> (w5147:string)
                    n2832 = Concatenate Strings(w5136, w5161, w5138) -> (w5151:string)
                    n2833 = Concatenate Strings(w5137, w5162, w5138) -> (w5152:string)
                    n2834 = Concatenate Strings(w5152, w5151, w5150, w5149, w5148, w5143, w5144, w5145, w5146, w5147) -> (w5121:string)
                    n2835 = Concatenate Strings("[PANEL/", "DESC/", "CYCLES/", "MINS/", "STATUS]", "\r", w5121) -> (w5120:string)
                    "MAIL REPORT" <- w5120
                    n2836 = global write "Global display 3.vi" "log all"(w5120) -> ()
                  }
                  frame #2 {
                    w5251 = "END"
                    n2837 = local read "mail control"() -> (w5252:string)
                    n2838 = case shown="False" w5247 {
                      tunnel: w5252 -> [w5276 _]
                      tunnel: w5251 -> [w5275 _]
                      tunnel: [w5274 FALSE] -> w5237
                      frame False {
                        n2839 = Equal?(x=w5276, y=w5275) -> (x = y?=w5274:bool)
                      }
                      frame True {
                      }
                    }
                    n2840 = case shown="False" w5253 {
                      tunnel: w5252 -> [w5292 _]
                      tunnel: w5251 -> [w5291 _]
                      tunnel: [w5290 FALSE] -> w5241
                      frame False {
                        n2841 = Equal?(x=w5292, y=w5291) -> (x = y?=w5290:bool)
                      }
                      frame True {
                      }
                    }
                    n2842 = case shown="False" w5250 {
                      tunnel: w5252 -> [w5288 _]
                      tunnel: w5251 -> [w5287 _]
                      tunnel: [w5286 FALSE] -> w5240
                      frame False {
                        n2843 = Equal?(x=w5288, y=w5287) -> (x = y?=w5286:bool)
                      }
                      frame True {
                      }
                    }
                    n2844 = case shown="False" w5248 {
                      tunnel: w5252 -> [w5280 _]
                      tunnel: w5251 -> [w5279 _]
                      tunnel: [w5278 FALSE] -> w5238
                      frame False {
                        n2845 = Equal?(x=w5280, y=w5279) -> (x = y?=w5278:bool)
                      }
                      frame True {
                      }
                    }
                    n2846 = case shown="False" w5249 {
                      tunnel: w5252 -> [w5284 _]
                      tunnel: w5251 -> [w5283 _]
                      tunnel: [w5282 FALSE] -> w5239
                      frame False {
                        n2847 = Equal?(x=w5284, y=w5283) -> (x = y?=w5282:bool)
                      }
                      frame True {
                      }
                    }
                    n2848 = Or(x=w5239, y=w5238) -> (x .or. y?=w5230:bool)
                    n2849 = Or(x=w5241, y=w5240) -> (x .or. y?=w5231:bool)
                    n2850 = Or(x=w5231, y=w5230) -> (x .or. y?=w5226:bool)
                    n2851 = case shown="False" w5243 {
                      tunnel: w5252 -> [w5260 _]
                      tunnel: w5251 -> [w5259 _]
                      tunnel: [w5258 FALSE] -> w5232
                      frame False {
                        n2852 = Equal?(x=w5260, y=w5259) -> (x = y?=w5258:bool)
                      }
                      frame True {
                      }
                    }
                    n2853 = case shown="False" w5242 {
                      tunnel: w5252 -> [w5256 _]
                      tunnel: w5251 -> [w5255 _]
                      tunnel: [w5254 FALSE] -> w5236
                      frame False {
                        n2854 = Equal?(x=w5256, y=w5255) -> (x = y?=w5254:bool)
                      }
                      frame True {
                      }
                    }
                    n2855 = case shown="False" w5244 {
                      tunnel: w5252 -> [w5264 _]
                      tunnel: w5251 -> [w5263 _]
                      tunnel: [w5262 FALSE] -> w5233
                      frame False {
                        n2856 = Equal?(x=w5264, y=w5263) -> (x = y?=w5262:bool)
                      }
                      frame True {
                      }
                    }
                    n2857 = case shown="False" w5246 {
                      tunnel: w5252 -> [w5272 _]
                      tunnel: w5251 -> [w5271 _]
                      tunnel: [w5270 FALSE] -> w5235
                      frame False {
                        n2858 = Equal?(x=w5272, y=w5271) -> (x = y?=w5270:bool)
                      }
                      frame True {
                      }
                    }
                    n2859 = case shown="False" w5245 {
                      tunnel: w5252 -> [w5268 _]
                      tunnel: w5251 -> [w5267 _]
                      tunnel: [w5266 FALSE] -> w5234
                      frame False {
                        n2860 = Equal?(x=w5268, y=w5267) -> (x = y?=w5266:bool)
                      }
                      frame True {
                      }
                    }
                    n2861 = Or(x=w5235, y=w5234) -> (x .or. y?=w5229:bool)
                    n2862 = Or(x=w5233, y=w5232) -> (x .or. y?=w5228:bool)
                    n2863 = Or(x=w5236, y=w5237) -> (x .or. y?=w5224:bool)
                    n2864 = Or(x=w5229, y=w5228) -> (x .or. y?=w5227:bool)
                    n2865 = Or(x=w5226, y=w5227) -> (x .or. y?=w5225:bool)
                    n2866 = Or(x=w5225, y=w5224) -> (x .or. y?=w5223:bool)
                  }
                  frame #3 {
                    n2867 = local read "on loops"() -> (w5306:dbl)
                    n2868 = local read "jig cycle"() -> (w5303:dbl)
                    n2869 = local read "Send Mail Now"() -> (w5297:bool)
                    n2870 = Add(x=w5306, y=3.0) -> (x+y=w5304:dbl)
                    n2871 = Equal?(x=w5303, y=w5304) -> (x = y?=w5298:bool)
                    n2872 = And(x=w5298, y=w5297) -> (x .and. y?=w5296:bool)
                    n2873 = And(x=w5302, y=w5298) -> (x .and. y?=w5301:bool)
                    n2874 = And(x=w5301, y=w5300) -> (x .and. y?=w5299:bool)
                    n2875 = Or(x=w5299, y=w5296) -> (x .or. y?=w5295:bool)
                    n2876 = case shown="True" w5295 {
                      tunnel: w5311 -> [_ w5317]
                      tunnel: w5310 -> [_ w5316]
                      tunnel: "Lab Panel Test Status" -> [_ w5315]
                      tunnel: w5308 -> [_ w5314]
                      tunnel: w5307 -> [_ w5313]
                      tunnel: w5294 -> [_ w5312]
                      frame False {
                      }
                      frame True {
                        n2877 = stacked-sequence {
                          tunnel: w5317 -> [w5325 _]
                          tunnel: w5316 -> [w5324 _]
                          tunnel: w5315 -> [w5323 _]
                          tunnel: w5314 -> [w5322 _]
                          tunnel: w5313 -> [w5321 _]
                          tunnel: w5312 -> [w5320 _]
                          frame #0 {
                            n2878 = call "sub vi - send mail v5.vi"("TO:"=w5325, "subject"=w5323, "from"=w5321, "out going server"=w5322, "message"=w5324) -> ("error out"=w5319:errorcluster)  [unwired: 10 in]
                            n2879 = Bundle(cluster=w5320, "mail error"=w5319) -> (w5318:T7)  [unwired: 6 in]
                            n2880 = local write "MAIL SETTINGS"(w5318) -> ()
                          }
                          frame #1 {
                            n2881 = local write "mail control"("") -> ()
                            n2882 = local write "Send Mail Now"(FALSE) -> ()
                          }
                        }
                      }
                    }
                  }
                }
              }
            }
          }
          frame #18 {
            # "save jig cycle values once all run switches are off"
            n2883 = stacked-sequence {
              tunnel: w5337 -> [_ w5366]
              tunnel: w5336 -> [_ w5365]
              tunnel: w5335 -> [_ w5364]
              tunnel: w5334 -> [_ w5363]
              tunnel: w5333 -> [_ w5362]
              tunnel: w5332 -> [_ w5361]
              tunnel: w5331 -> [_ w5360]
              tunnel: w5330 -> [_ w5359]
              tunnel: w5329 -> [_ w5358]
              tunnel: w5328 -> [_ w5357]
              frame #0 {
              }
              frame #1 {
                n2884 = Not(x=w5357) -> (.not. x?=w5340:bool)
                n2885 = Not(x=w5365) -> (.not. x?=w5355:bool)
                n2886 = Not(x=w5362) -> (.not. x?=w5350:bool)
                n2887 = Not(x=w5360) -> (.not. x?=w5346:bool)
                n2888 = Not(x=w5358) -> (.not. x?=w5342:bool)
                n2889 = Not(x=w5366) -> (.not. x?=w5356:bool)
                n2890 = Not(x=w5364) -> (.not. x?=w5354:bool)
                n2891 = Not(x=w5361) -> (.not. x?=w5348:bool)
                n2892 = Not(x=w5363) -> (.not. x?=w5352:bool)
                n2893 = Not(x=w5359) -> (.not. x?=w5344:bool)
                n2894 = local read "Save JC"() -> (w5368:bool)
                n2895 = And(x=w5356, y=w5355) -> (x .and. y?=w5353:bool)
                n2896 = And(x=w5353, y=w5354) -> (x .and. y?=w5351:bool)
                n2897 = And(x=w5351, y=w5352) -> (x .and. y?=w5349:bool)
                n2898 = And(x=w5349, y=w5350) -> (x .and. y?=w5347:bool)
                n2899 = And(x=w5347, y=w5348) -> (x .and. y?=w5345:bool)
                n2900 = And(x=w5345, y=w5346) -> (x .and. y?=w5343:bool)
                n2901 = And(x=w5343, y=w5344) -> (x .and. y?=w5341:bool)
                n2902 = And(x=w5341, y=w5342) -> (x .and. y?=w5339:bool)
                n2903 = And(x=w5339, y=w5340) -> (x .and. y?=w5338:bool)
                n2904 = And(x=w5338, y=w5368) -> (x .and. y?=w5367:bool)
                n2905 = case shown="True" w5367 {
                  tunnel: w5338 -> [w5369 _]
                  frame False {
                    n2906 = case shown="False" w5369 {
                      frame False {
                        n2907 = local write "Save JC"(TRUE) -> ()
                      }
                      frame True {
                      }
                    }
                  }
                  frame True {
                    n2908 = stacked-sequence {
                      frame #0 {
                        n2909 = String To Path(string="c:\\crabtree\\Jig Cycles\\") -> (path=w5381:path)
